vi "CRYClose All Graph.vi"(11 "DataView Array Idx In":i32) -> ()   [LabVIEW 2013]
uses:
  CRYNew View Global.vi
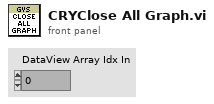
[diagram p1: front panel]
types:
  T1 = typedef "Graph Main Info Cluster.ctl" = cluster{"Selected_BarIdx":i32, "Selected_PanelIdx":i32, "Graph Main VIRef":refnum<vi>, "ToolBarClick":bool, "Spliter Ref Array":refnum<vi>[], "Panel Ref Array":refnum<vi>[], "Spliter_matrix":i32[][], "Panel_matrix":i32[][], "child_spliterIdx_matrix":i32[][], "split_pos_matrix":i32[][], "Title State":bool, "sQueueName":string, "Frame nID":i32, "Graph VIRef Array":cluster{"Graph VIRef":refnum<vi>, "Panel Idx":i32, "Frame VIRef":refnum<vi>, "Icon Ring":i32, "Graph Type":string}[], "View Type":string}
  T2 = cluster{"Graph VIRef":refnum<vi>, "Panel Idx":i32, "Frame VIRef":refnum<vi>, "Icon Ring":i32, "Graph Type":string}[]
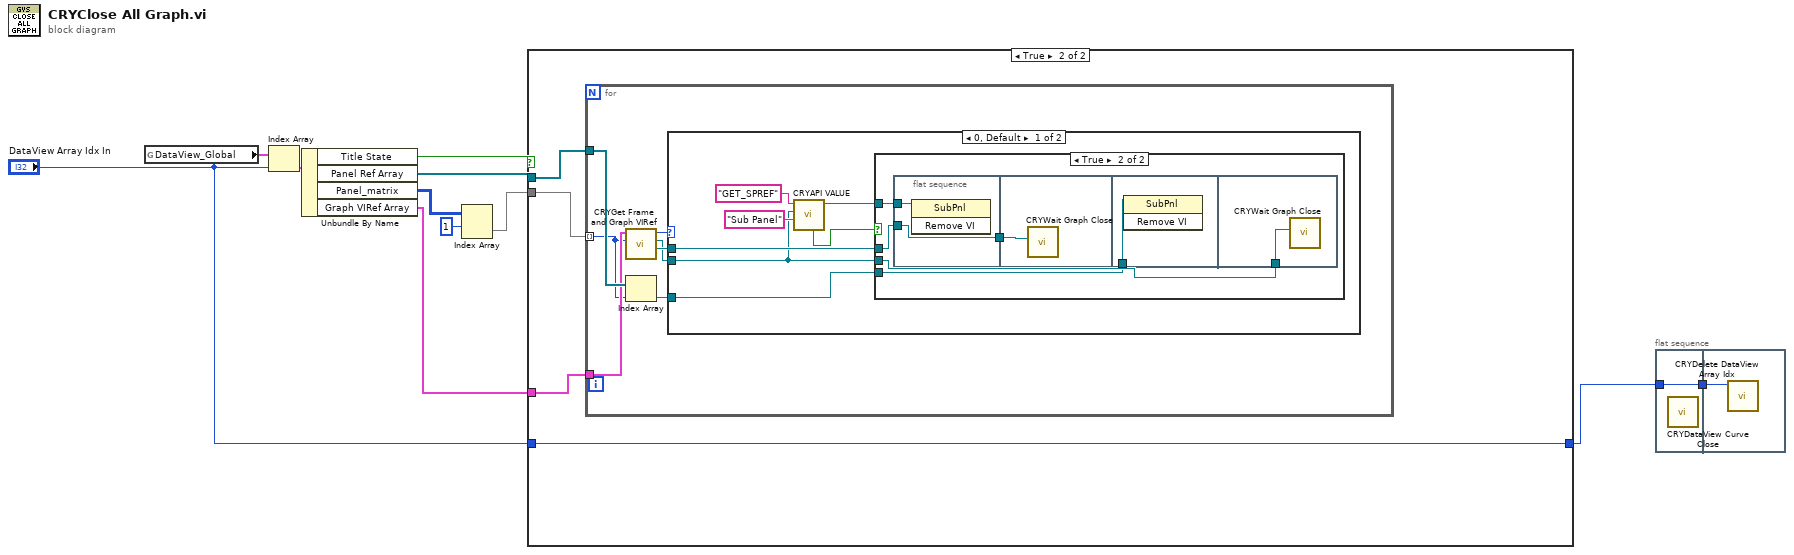
[diagram p0: block diagram]
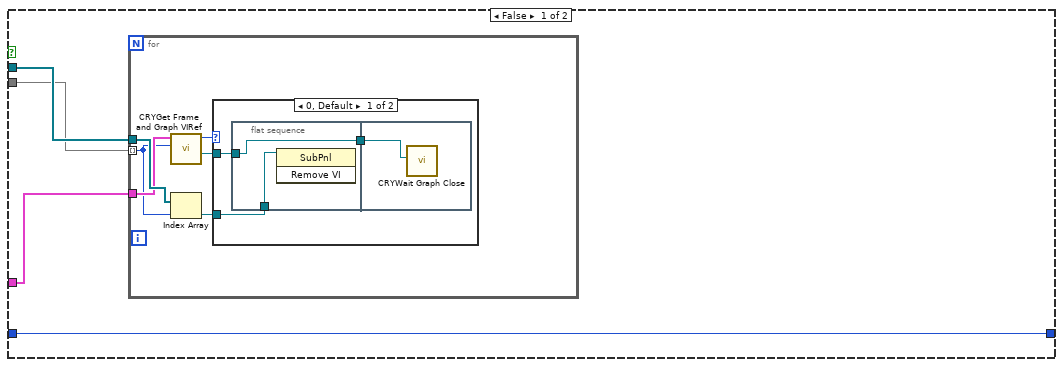
[diagram p2: hidden frame]
diagram:
  n1 = global read "CRYNew View Global.vi" "DataView_Global"() -> (w11:T1[])
  n2 = Index Array(array=w11, index="DataView Array Idx In") -> (element=w10:T1)
  n3 = Unbundle By Name(w10) -> ("Title State"=w9:bool, "Panel Ref Array"=w8:refnum<vi>[], "Panel_matrix"=w6:i32[][], "Graph VIRef Array"=w3:T2)
  n4 = Index Array(array=w6, index (row)=1) -> (element=w4:i32[])  [unwired: 1 in]
  n5 = case shown="True" w9 {
    tunnel: w8 -> [w15 w30]
    tunnel: "DataView Array Idx In" -> [w14 w31]
    tunnel: [w14 w31] -> w2
    tunnel: w4 -> [w13 w29]
    tunnel: w3 -> [w12 w28]
    frame False {
      n6 = for {
        tunnel: w15 -> [w21]
        tunnel: w13 -> [w19] mode=indexing
        tunnel: w12 -> [w20]
        n7 = call "CRYGet Frame and Graph VIRef.vi"("Panel Idx"=w19, "Graph VIRef Array"=w20) -> ("Graph VIRef"=w17:refnum<vi>, "Graph VIRef Array Index"=w18:i32)  [unwired: 5 in, 3 out]
        n8 = Index Array(array=w21, index=w19) -> (element=w16:refnum<vi>)
        n9 = case shown="0, Default" w18 {
          tunnel: w17 -> [w24 _]
          tunnel: w16 -> [w23 _]
          frame 0, Default {
            n10 = flat-sequence {
              tunnel: w24 -> [w25]
              tunnel: w23 -> [w26]
              tunnel: [w25] -> w22
              tunnel: w22 -> [w27]
              frame #0 {
                n11 = invoke class="SubPnl" method="Remove VI"(reference=w26) -> ()  [unwired: 2 in, 3 out]
              }
              frame #1 {
                n12 = call "CRYWait Graph Close.vi"("vi reference"=w27) -> ()  [unwired: 11 in]
              }
            }
          }
          frame -1 {
          }
        }
      }
    }
    frame True {
      n13 = for {
        tunnel: w30 -> [w38]
        tunnel: w29 -> [w36] mode=indexing
        tunnel: w28 -> [w37]
        n14 = call "CRYGet Frame and Graph VIRef.vi"("Panel Idx"=w36, "Graph VIRef Array"=w37) -> ("Graph VIRef"=w34:refnum<vi>, "Frame VIRef"=w33:refnum<vi>, "Graph VIRef Array Index"=w35:i32)  [unwired: 5 in, 2 out]
        n15 = Index Array(array=w38, index=w36) -> (element=w32:refnum<vi>)
        n16 = case shown="0, Default" w35 {
          tunnel: w34 -> [w45 _]
          tunnel: w33 -> [w41 _]
          tunnel: w32 -> [w39 _]
          frame 0, Default {
            n17 = call "CRYAPI VALUE.vi"("sControlName"="Sub Panel", "pVIRef"=w41, "sAction"="GET_SPREF") -> ("pSPRef"=w40:refnum<vi>, "bResult"=w42:bool)  [unwired: 2 in, 5 out]
            n18 = case shown="True" w42 {
              tunnel: w45 -> [_ w50]
              tunnel: w41 -> [_ w47]
              tunnel: w40 -> [_ w49]
              tunnel: w39 -> [_ w46]
              frame False {
              }
              frame True {
                n19 = flat-sequence {
                  tunnel: w50 -> [w51]
                  tunnel: w49 -> [w52]
                  tunnel: [w51] -> w48
                  tunnel: w48 -> [w53]
                  tunnel: w46 -> [w54]
                  tunnel: w47 -> [w55]
                  frame #0 {
                    n20 = invoke class="SubPnl" method="Remove VI"(reference=w52) -> ()  [unwired: 2 in, 3 out]
                  }
                  frame #1 {
                    n21 = call "CRYWait Graph Close.vi"("vi reference"=w53) -> ()  [unwired: 11 in]
                  }
                  frame #2 {
                    n22 = invoke class="SubPnl" method="Remove VI"(reference=w54) -> ()  [unwired: 2 in, 3 out]
                  }
                  frame #3 {
                    n23 = call "CRYWait Graph Close.vi"("vi reference"=w55) -> ()  [unwired: 11 in]
                  }
                }
              }
            }
          }
          frame -1 {
          }
        }
      }
    }
  }
  n24 = flat-sequence {
    tunnel: w2 -> [w56]
    tunnel: [w56] -> w1
    tunnel: w1 -> [w57]
    frame #0 {
      n25 = call "CRYDataView Curve Close.vi"() -> ()  [unwired: 12 in]
    }
    frame #1 {
      n26 = call "CRYDelete DataView Array Idx.vi"("DataView Idx In"=w57) -> ()  [unwired: 11 in]
    }
  }
